vi "Controllers_PIDPiezoReset.vi"(8 "PID ON/OFF IN":bool, 9 "PID ON/OFF [i-1]":bool, 11 "Piezo V":dbl) -> (3 "Piezo V":dbl)   [LabVIEW 2023]
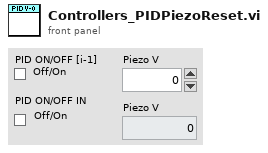
[diagram p1: front panel]
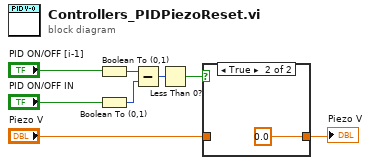
[diagram p0: block diagram]
diagram:
  n1 = Boolean To (0,1)(Boolean="PID ON/OFF [i-1]") -> (0, 1=w8:i16)
  n2 = Boolean To (0,1)(Boolean="PID ON/OFF IN") -> (0, 1=w7:i16)
  n3 = Subtract(x=w8, y=w7) -> (x-y=w6:i16)
  n4 = Less Than 0?(x=w6) -> (x < 0?=w5:bool)
  n5 = case shown="True" w5 {
    tunnel: [w9 0.0] -> w4
    tunnel: "Piezo V" -> [w9 _]
    frame False {
    }
    frame True {
    }
  }
  "Piezo V" <- w4
